vi "Pre Launch Init.vi"(11 "Simulated User Console Actor in":refnum<class "Simulated Sensor Interface Actor.lvclass">) -> (0 "error out":errorcluster, 3 "Simulated User Console Actor out":refnum<class "Simulated Sensor Interface Actor.lvclass">)   [LabVIEW 2019, in "Simulated Sensor Interface Actor.lvlib" / "Simulated Sensor Interface Actor.lvclass"]
doc: "(<B>Filename</B>: Actor Framework.lvlib:Actor.lvclass:Pre Launch Init.vi)\n\nDefines behavior that occurs after the Launch Nested Actor method is invoked but before the actor's Actor Core method begins running.\n\nBy default, this method does nothing. A descendant class may override it to define behavior."
uses:
  Simulated Sensor Interface Actor.lvclass
  Simulated Sensor Interface Actor.lvclass/Simulated Sensor Interface Actor.ctl
  Sensor Interface Actor/Sensor Interface Actor/Sensor Interface Actor.lvclass
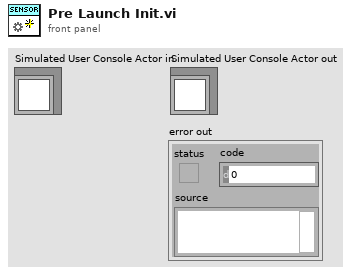
[diagram p1: front panel]
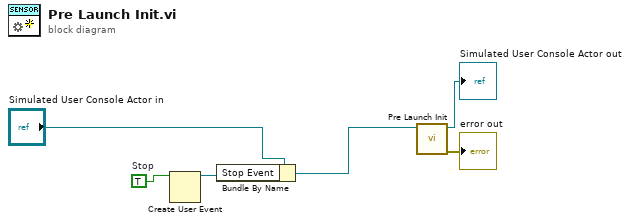
[diagram p0: block diagram]
diagram:
  w4 = TRUE  # Stop
  n1 = Create User Event(user event datatype=w4) -> (user event=w2:refnum<user-event>)  [unwired: 1 in, 1 out]
  n2 = Bundle By Name(cluster="Simulated User Console Actor in", "Stop Event"=w2) -> (w1:refnum<class "Simulated Sensor Interface Actor.lvclass">)
  n3 = call-parent "Pre Launch Init.vi"("Actor in"=w1) -> ("error out"=→"error out":errorcluster, "Actor out"=→"Simulated User Console Actor out":refnum<class "Simulated Sensor Interface Actor.lvclass">)  [unwired: 9 in]
